vi "Greatek.vi"(8 "error in (no error)":errorcluster, 9 "Boolean":bool, 10 "name or relative path":string="libvlc.dll", 11 ".NET Refnum in":refnum<k24>(container)) -> (0 "error out":errorcluster)   [LabVIEW 2018]
uses:
  System.Windows.Forms
panel:
  out "error out 2":errorcluster
  out "return type":i32
  out "p_mi":i32
  out "path out":path
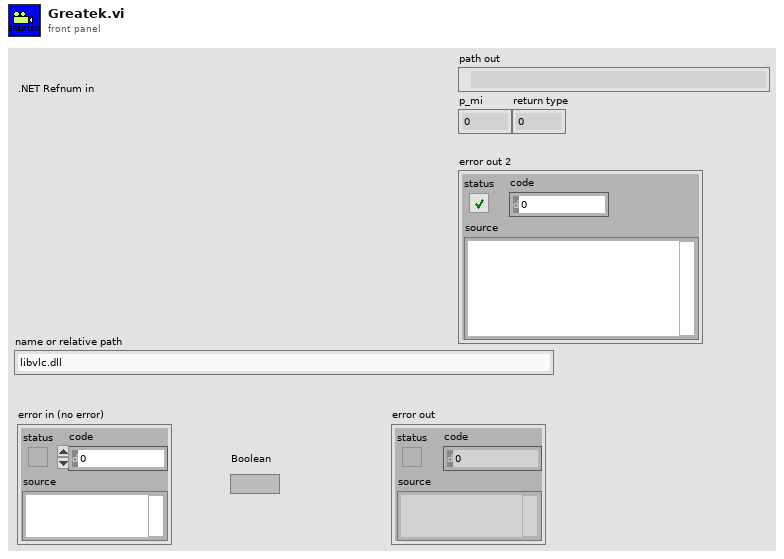
[diagram p1: front panel]
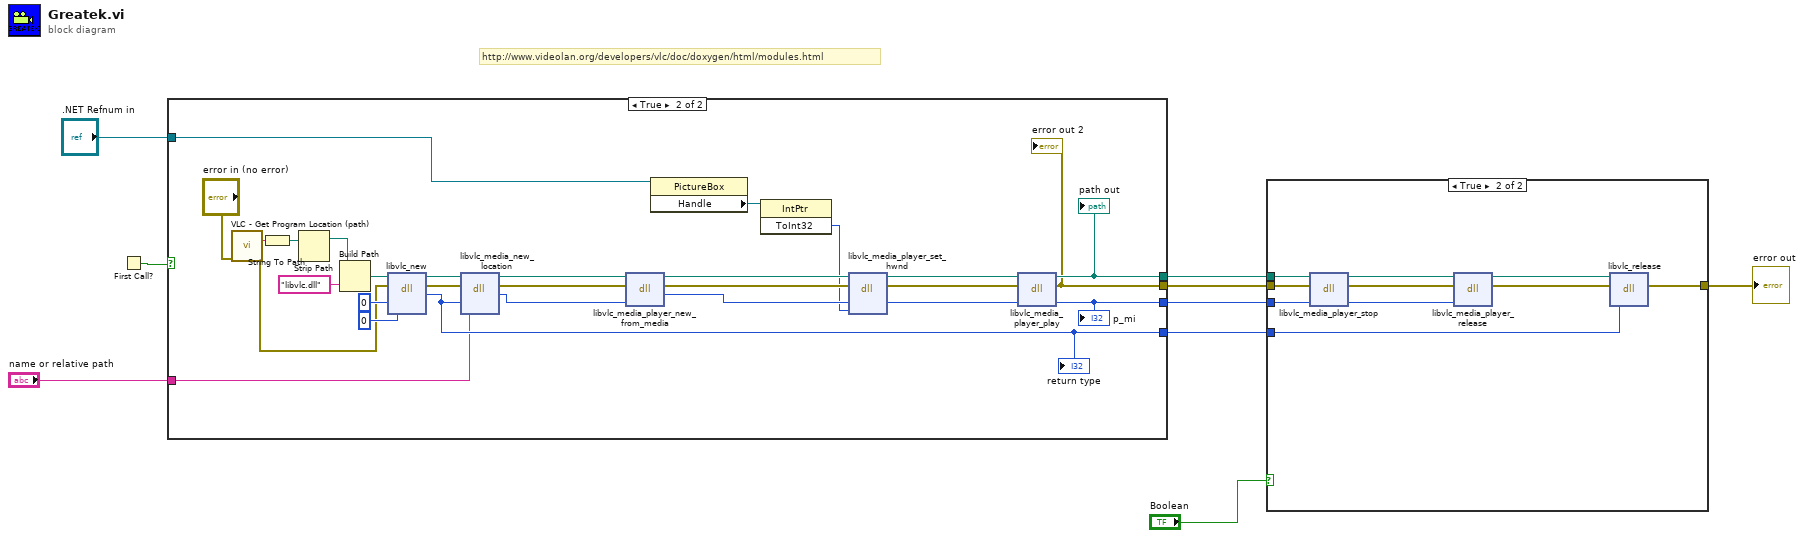
[diagram p0: block diagram]
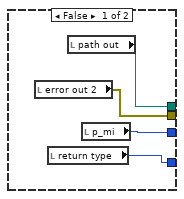
[diagram p3: hidden frame]
diagram:
  # "http://www.videolan.org/developers/vlc/doc/doxygen/html/modules.html"
  n1 = First Call?() -> (First Call?: T/F=w9:bool)
  n2 = case shown="True" w9 {
    tunnel: [w13 w41] -> w3
    tunnel: [w12 w40] -> w4
    tunnel: [w11 w29] -> w5
    tunnel: "name or relative path" -> [_ w23]
    tunnel: [w10 w20] -> w7
    tunnel: ".NET Refnum in" -> [_ w18]
    frame False {
      n3 = local read "error out 2"() -> (w10:errorcluster)
      n4 = local read "return type"() -> (w13:i32)
      n5 = local read "path out"() -> (w11:path)
      n6 = local read "p_mi"() -> (w12:i32)
    }
    frame True {
      n7 = call "VLC - Get Program Location (path).vi"("error in (no error)"="error in (no error)") -> ("VLC path"=w28:string, "error out"=w21:errorcluster)  [unwired: 13 in]
      n8 = String To Path(string=w28) -> (path=w27:path)
      n9 = Strip Path(path=w27) -> (stripped path=w26:path)  [unwired: 1 out]
      n10 = Build Path(base path=w26, name or relative path="libvlc.dll") -> (appended path=w24:path)
      n11 = dll-call lib="C:/Program Files (x86)/VideoLAN/VLC/libvlc.dll" fn="libvlc_new"(path in=w24, error in=w21, "argc"=i16 0, "argv"=u8 0) -> (path out=w32:path, error out=w35:errorcluster, "return type"=w41:i32)  [unwired: 3 in]
      "return type" <- w41
      n12 = dll-call lib="C:/Program Files (x86)/VideoLAN/VLC/libvlc.dll" fn="libvlc_media_new_location"(path in=w32, error in=w35, "p_instance"=w41, "path"=w23) -> (path out=w19:path, error out=w15:errorcluster, "return type"=w14:i32)  [unwired: 3 in]
      n13 = dll-call lib="C:/Program Files (x86)/VideoLAN/VLC/libvlc.dll" fn="libvlc_media_player_new_from_media"(path in=w19, error in=w15, "p_md"=w14) -> (path out=w31:path, error out=w38:errorcluster, "return type"=w36:i32)  [unwired: 2 in]
      n14 = property class="PictureBox"(reference=w18) -> ("Handle"=w17:refnum<k24>)  [unwired: 1 in, 2 out]
      n15 = invoke class="IntPtr" method="ToInt32"(reference=w17) -> ("ToInt32"=w16:i32)  [unwired: 2 in, 2 out]
      n16 = dll-call lib="C:/Program Files (x86)/VideoLAN/VLC/libvlc.dll" fn="libvlc_media_player_set_hwnd"(path in=w31, error in=w38, "p_mi"=w36, "drawable"=w16) -> (path out=w30:path, error out=w39:errorcluster, "p_mi"=w37:i32)  [unwired: 3 in]
      n17 = dll-call lib="C:/Program Files (x86)/VideoLAN/VLC/libvlc.dll" fn="libvlc_media_player_play"(path in=w30, error in=w39, "p_mi"=w37) -> (path out=w29:path, error out=w20:errorcluster, "p_mi"=w40:i32)  [unwired: 2 in]
      "path out" <- w29
      "p_mi" <- w40
      "error out 2" <- w20
    }
  }
  n18 = case shown="True" "Boolean" {
    tunnel: w7 -> [w42 w52]
    tunnel: [w42 w51] -> w6
    tunnel: w5 -> [_ w50]
    tunnel: w4 -> [_ w49]
    tunnel: w3 -> [_ w48]
    frame False {
    }
    frame True {
      n19 = dll-call lib="C:/Program Files (x86)/VideoLAN/VLC/libvlc.dll" fn="libvlc_media_player_stop"(path in=w50, error in=w52, "p_mi"=w49) -> (path out=w44:path, error out=w47:errorcluster, "p_mi"=w46:i32)  [unwired: 2 in]
      n20 = dll-call lib="C:/Program Files (x86)/VideoLAN/VLC/libvlc.dll" fn="libvlc_media_player_release"(path in=w44, error in=w47, "p_mi"=w46) -> (path out=w43:path, error out=w45:errorcluster)  [unwired: 3 in]
      n21 = dll-call lib="C:/Program Files (x86)/VideoLAN/VLC/libvlc.dll" fn="libvlc_release"(path in=w43, error in=w45, "p_instnace"=w48) -> (error out=w51:errorcluster)  [unwired: 3 in, 1 out]
    }
  }
  "error out" <- w6
